vi "Run Panel.vi"(8 "error in (no error)":errorcluster, 10 "Panel In":refnum<class "Panel.lvclass">, 11 "Manager in":refnum<class "Manager.lvclass">) -> (0 "error out":errorcluster, 2 "Panel":refnum<class "Panel.lvclass">, 3 "Manager out":refnum<class "Manager.lvclass">)   [LabVIEW 2020, in "OOPanel.lvlib" / "Manager.lvclass"]
uses:
  Manager.lvclass
  Panel/Panel.lvclass
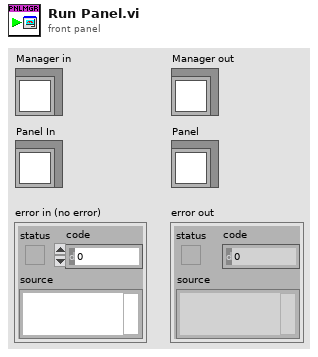
[diagram p1: front panel]
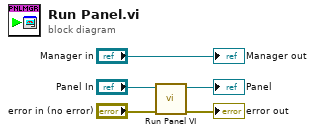
[diagram p0: block diagram]
diagram:
  n1 = call "Run Panel VI.vi"("error in (no error)"="error in (no error)", "Panel in"="Panel In") -> ("error out"=→"error out":errorcluster, "Panel out"=→"Panel":refnum<class "Panel.lvclass">)  [unwired: 8 in]
  "Manager out" <- "Manager in"
